vi "NXTLineLeader-Direct.vi"() -> ()   [LabVIEW 2009]
uses:
  <vilib>/NXT/Block Support/NXT_InputPort.ctl
  <vilib>/NXT/Subs/LVHSConnector.ctl
panel:
  out "NXT dup":T1={"error"={"status"=FALSE, "code"=0, "source"=""}, "address"="", "NXT #"=-1, "Show Error"=TRUE}
  in  "NXT":T1={"error"={"status"=FALSE, "code"=0, "source"=""}, "address"="", "NXT #"=-1, "Show Error"=TRUE}
  out "?":bool[](array[boolean])
  out "Sensor 8 Reading":u8
  out "Sensor 7 Reading":u8
  out "Sensor 6 Reading":u8
  out "Sensor 5 Reading":u8
  out "Sensor 4 Reading":u8
  out "Sensor 3 Reading":u8
  out "Sensor 2 Reading":u8
  out "Sensor 1 Reading":u8
  in  "Select your \nInput Port":T2 items=["Port 1", "Port 2", "Port 3", "Port 4"]
  in  "?":bool=TRUE
  # "mindsensors.com\nCopyright (c) 2009 by mindsensors.com\nEmail: info (<at>) mindsensors (<dot>) com\n\nThis program is free software. You can redistribute it and/or modify\nit under the terms of the GNU General Public License as published by\nthe Free Software Foundation; version 3 of the License.\nRead the license at: http://www.gnu.org/licenses/gpl.txt"
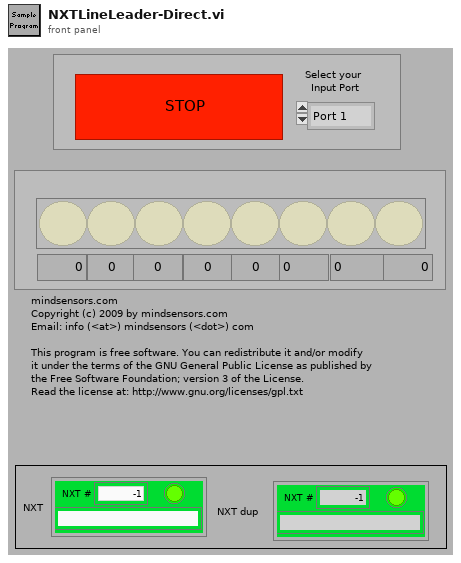
[diagram p1: front panel]
types:
  T1 = typedef "LVHSConnector.ctl" = cluster{"error":errorcluster, "address":string, "NXT #":i32, "Show Error":bool}
  T2 = typedef "NXT_InputPort.ctl" = u8
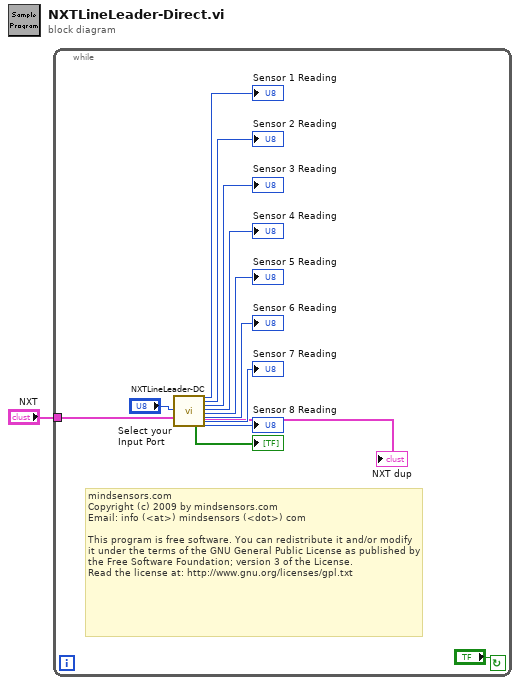
[diagram p0: block diagram]
diagram:
  n1 = while {
    tunnel: "NXT" -> [w3]
    stop <- "?" continue-if-true
    # "mindsensors.com\nCopyright (c) 2009 by mindsensors.com\nEmail: info (<at>) mindsensors (<dot>) com\n\nThis program is free software. You can redistribute it and/or modify\nit under the terms of the GNU General Public License as published by\nthe Free Software Foundation; version 3 of the License.\nRead the license at: http://www.gnu.org/licenses/gpl.txt"
    n2 = call "NXTLineLeader-DC.vi"("Select your \nInput Port"="Select your \nInput Port", "NXT"=w3) -> ("Boolean array"=→"?":bool[], "NXT dup"=→"NXT dup":T1, "Sensor 1 Reading"=→"Sensor 1 Reading":u8, "Sensor 2 Reading"=→"Sensor 2 Reading":u8, "Sensor 3 Reading"=→"Sensor 3 Reading":u8, "Sensor 4 Reading"=→"Sensor 4 Reading":u8, "Sensor 5 Reading"=→"Sensor 5 Reading":u8, "Sensor 6 Reading"=→"Sensor 6 Reading":u8, "Sensor 7 Reading"=→"Sensor 7 Reading":u8, "Sensor 8 Reading"=→"Sensor 8 Reading":u8)  [unwired: 16 in]
  }
